vi "Region-det-Q-gen-util.vi"(8 "error in":errorcluster, 10 "Actual Q matrix JSON - rel path":path=path "../traffic_1_dict.json", 11 "Q matrix info JSON - rel path":path=path "../traffic_1_size_dict.json") -> (0 "error out":errorcluster, 1 "Q Matrices":dbl[][][][](array[numeric]), 2 "Index array":dbl[](array[numeric]), 3 "Regions":i32[](array[numeric]))   [LabVIEW 2016]
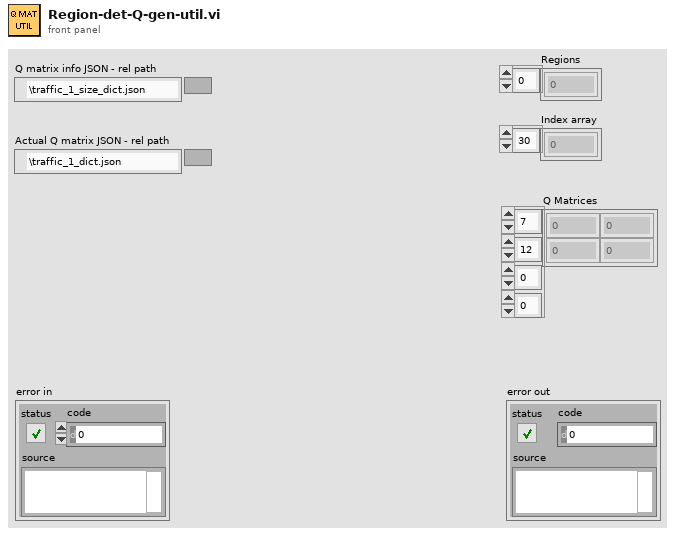
[diagram p1: front panel]
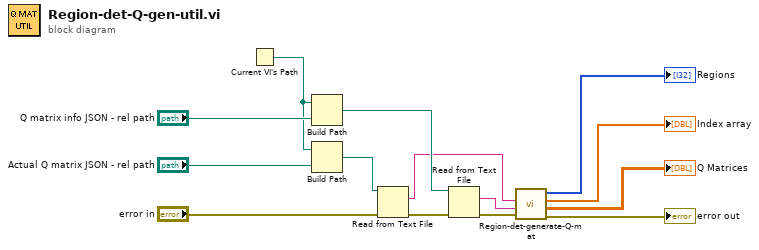
[diagram p0: block diagram]
diagram:
  n1 = Current VI's Path() -> (path=w10:path)
  n2 = Build Path(base path=w10, name or relative path="Q matrix info JSON - rel path") -> (appended path=w11:path)
  n3 = Build Path(base path=w10, name or relative path="Actual Q matrix JSON - rel path") -> (appended path=w14:path)
  n4 = Read from Text File(file (use dialog)=w14, error in="error in") -> (text=w7:string, error out=w9:errorcluster)  [unwired: 2 in, 2 out]
  n5 = Read from Text File(file (use dialog)=w11, error in=w9) -> (text=w6:string, error out=w5:errorcluster)  [unwired: 2 in, 2 out]
  n6 = call "Region-det-generate-Q-mat.vi"("error in (no error)"=w5, "Q region size JSON string"=w6, "Q matrix JSON string"=w7) -> ("error out"=→"error out":errorcluster, "Q Matrices"=→"Q Matrices":dbl[][][][], "Index array"=→"Index array":dbl[], "Regions"=→"Regions":i32[])  [unwired: 5 in]
